vi "Config Current Trip.vi"(0 "VISA resource name":refnum<visa-resource-name>, 7 "Trip Value (5.25 mA)":dbl=5.25 format="%.2f", 11 "error in (no error)":errorcluster) -> (4 "VISA resource name out":refnum<visa-resource-name>, 15 "error out":errorcluster)   [LabVIEW 2013, in "Stanford Research PS300 Series.lvlib"]
doc: "This VI sets the value for the current trip. The current trip shuts off the high voltage when the output current exceeds the trip value. \nAfter a current trip occurs, the 'ITRP' (current trip) message will appear in the middle display. \n\nNotes*: \n1) Voltage Trip: This may occur if the load changes too rapidly, causing the voltage to overshoot. A voltage trip message 'VTRP' will occur on the middle display. Try raising the voltage limit.\n\n2) Current Trip: Disconnect the load and see if the unit still trips. If it works with no load, there may be a problem with nthe load. If it still trips, the unit may be damaged. Please contact the factory for further information.\n \n3) Primary Trip: If repeated trips occur, the power supply may be damaged. Please contact the factory for further information. A primary trip message 'PTRP' will occur if the current through the primary side of the high voltage transformer and the switching MOSFET's exceeds about 5.3 Amps. This feature is included to protect the transformer and the FET's. The trip level is not user programmable"
uses:
  Stanford Research PS300 Series.lvlib
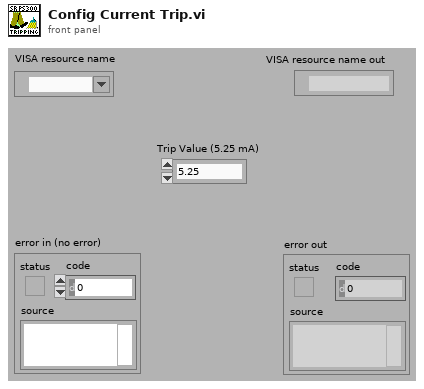
[diagram p1: front panel]
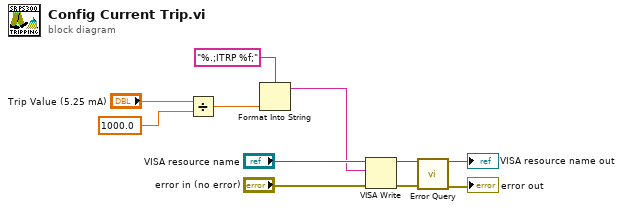
[diagram p0: block diagram]
diagram:
  n1 = Divide(x="Trip Value (5.25 mA)", y=1000.0) -> (x/y=w5:dbl)
  n2 = Format Into String(format string="%.;ITRP %f;", w5) -> (resulting string=w9:string)  [unwired: 2 in, 1 out]
  n3 = VISA Write(VISA resource name="VISA resource name", write buffer=w9, error in (no error)="error in (no error)") -> (VISA resource name out=w4:refnum<visa-resource-name>, error out=w3:errorcluster)  [unwired: 1 out]
  n4 = call "Error Query.vi"("VISA resource name"=w4, "error in (no error)"=w3) -> ("VISA resource name out"=→"VISA resource name out":refnum<visa-resource-name>, "error out"=→"error out":errorcluster)  [unwired: 10 in, 2 out]
